vi "Library Path_LLLB2.vi"(11 "File Path":path) -> (2 "Is in llb?":bool, 3 "llb path":path)   [LabVIEW 2023]
doc: "Determine if VI is in llb and retur llb path. Path out is empty if not llb."
uses:
  <userlib>/_OpenG.lib/file/file.llb/Strip Path Extension - String__ogtk.vi
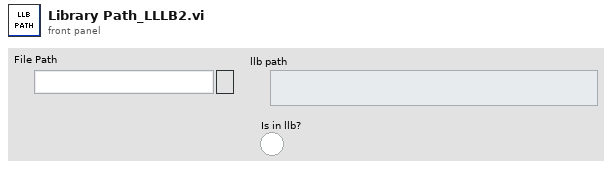
[diagram p1: front panel]
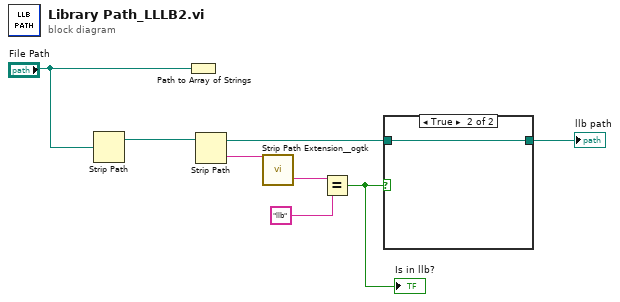
[diagram p0: block diagram]
diagram:
  n1 = Strip Path(path="File Path") -> (stripped path=w2:path)  [unwired: 1 out]
  n2 = Path to Array of Strings(0:"File Path") -> ()  [unwired: 2 out]
  n3 = Strip Path(path=w2) -> (stripped path=w5:path, name=w8:string)
  n4 = call-poly <userlib>:"Strip Path Extension__ogtk.vi"("path"=w8) -> ("extension"=w7:string)  [unwired: 1 out]
  n5 = Equal?(x=w7, y="llb") -> (x = y?=w1:bool)
  "Is in llb?" <- w1
  n6 = case shown="True" w1 {
    tunnel: [_ w9] -> w4
    tunnel: w5 -> [_ w9]
    frame False {
    }
    frame True {
    }
  }
  "llb path" <- w4
